vi "BLcompare.vi"(7 "Zref":dbl=500.0 min=0.0, 8 "Normalise?":bool=TRUE, 9 "aTarget":cluster{"Xvalues":dbl[], "Yvalues":dbl[]}={"Xvalues"=[0.75, 0.82, 0.85, 0.86, 0.9, 0.91, 0.94, 0.95, 0.96], "Yvalues"=[55.0, 75.0, 88.0, 122.0, 160.0, 220.0, 294.0, 385.0, 499.0]}, 10 "aSeries":cluster{"Xvalues":dbl[], "Yvalues":dbl[]}={"Xvalues"=[9.631456, 10.097028, 10.411531, 10.617216, 10.970124, 11.230059, 11.570385, 11.879879, 12.393209, 13.02907, 13.593284, 13.540779], "Yvalues"=[50.04624939, 67.04914093, 89.77313232, 120.27675629, 161.2066803, 216.03833008, 289.45019531, 387.77822876, 519.55065918, 696.23638916, 932.88671875, 1250.06018066]}) -> (0 "metric2value":dbl, 1 "metric2name":string, 2 "metric1value":dbl, 3 "metric1name":string)   [LabVIEW 2018]
uses:
  gnuplotScriptComponents/BLPlottersubVIs/Resampler.ctl
  <vilib>/Analysis/baseanly.llb/Mean (DBL).vi
  <vilib>/Analysis/5stat.llb/RMS (DBL).vi
  <vilib>/Analysis/NI_AALPro.lvlib
  <vilib>/Analysis/NI_AALBase.lvlib
panel:
  in  "BandHalfWidth(%)":dbl=0.05
  in  "Comparison":enum16{"PercentError", "PercentPointsInBand"}(ring)
  in  "milliseconds to wait":u32
  out "XY Graph":cluster{dbl[], dbl[]}[](graph)
  out "TargetResampled":cluster{"Xvalues":dbl[], "Yvalues":dbl[]}={"Xvalues"=[9.631456, 10.097028, 10.411531, 10.617216, 10.970124, 11.230059, 11.570385, 11.879879, 12.393209, 13.02907, 13.593284, 13.540779], "Yvalues"=[50.04624939, 67.04914093, 89.77313232, 120.27675629, 161.2066803, 216.03833008, 289.45019531, 387.77822876, 519.55065918, 696.23638916, 932.88671875, 1250.06018066]}
  out "aSeriesNormalised":cluster{"Xvalues":dbl[], "Yvalues":dbl[]}={"Xvalues"=[9.631456, 10.097028, 10.411531, 10.617216, 10.970124, 11.230059, 11.570385, 11.879879, 12.393209, 13.02907, 13.593284, 13.540779], "Yvalues"=[50.04624939, 67.04914093, 89.77313232, 120.27675629, 161.2066803, 216.03833008, 289.45019531, 387.77822876, 519.55065918, 696.23638916, 932.88671875, 1250.06018066]}
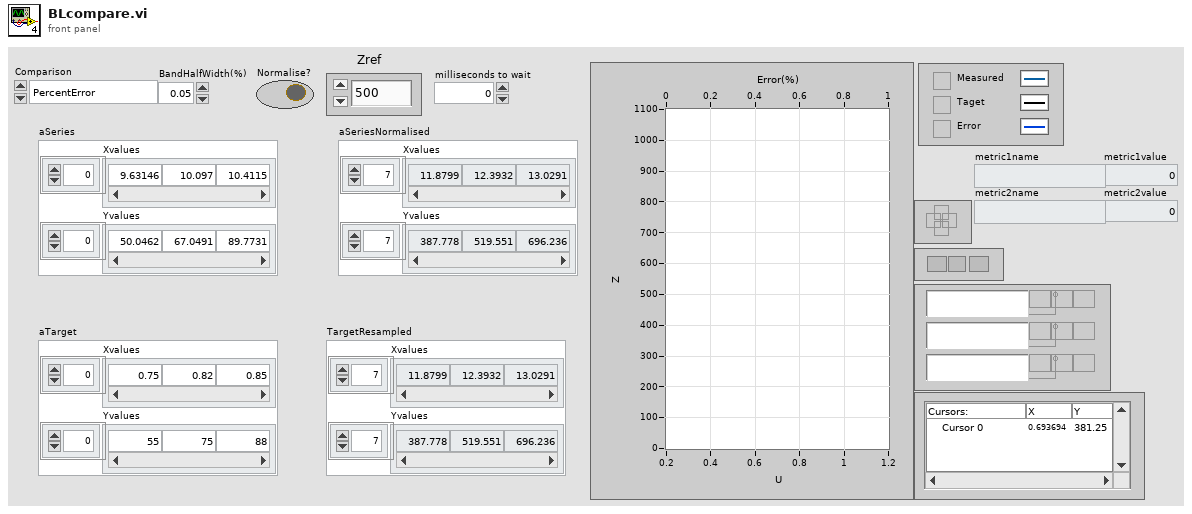
[diagram p1: front panel]
types:
  T1 = typedef "Resampler.ctl" = enum32{"AsTaken", "Regular", "Prescribed"}
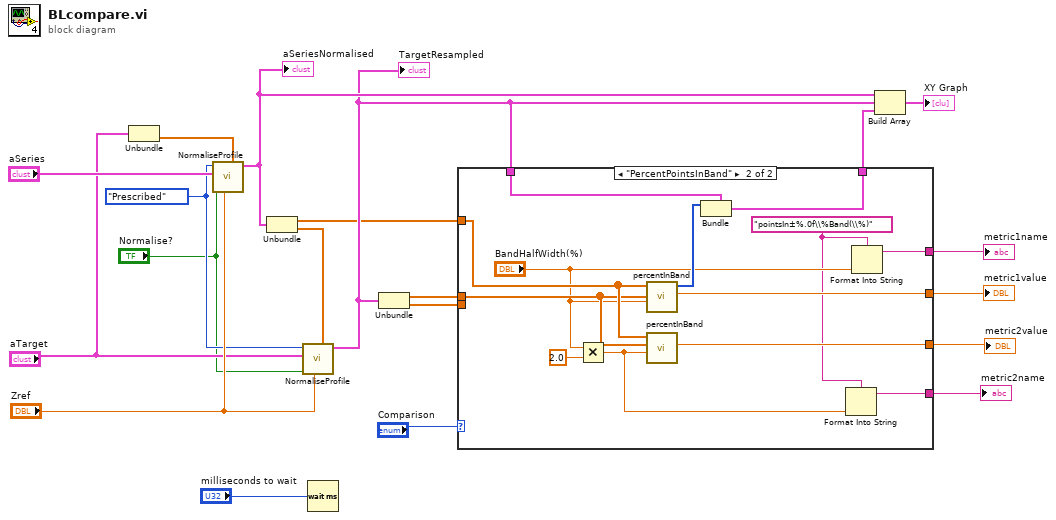
[diagram p0: block diagram]
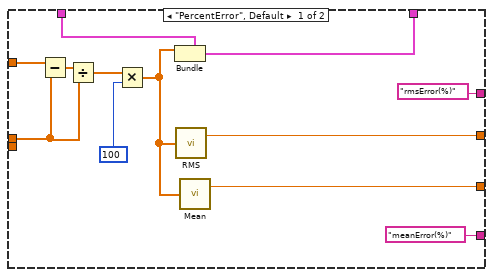
[diagram p2: hidden frame]
diagram:
  w15 = Resampler."Prescribed" ("Resampler")
  n1 = Unbundle("aTarget") -> ("Yvalues"=w16:dbl[])  [unwired: 1 out]
  n2 = call "NormaliseProfile.vi"("ResampleHeights"=w16, "Zref"="Zref", "Normalise?"="Normalise?", "UzClusterIn"="aSeries", "Resampler"=w15) -> ("UzClusterOutput"=w13:cluster{dbl[], dbl[]})  [unwired: 5 in, 1 out]
  "aSeriesNormalised" <- w13
  n3 = Unbundle(w13) -> (w9:dbl[], w19:dbl[])
  n4 = call "NormaliseProfile.vi"("ResampleHeights"=w19, "Zref"="Zref", "Normalise?"="Normalise?", "UzClusterIn"="aTarget", "Resampler"=w15) -> ("UzClusterOutput"=w12:cluster{dbl[], dbl[]})  [unwired: 5 in, 1 out]
  "TargetResampled" <- w12
  n5 = Wait (ms)(milliseconds to wait="milliseconds to wait") -> ()  [unwired: 1 out]
  n6 = Unbundle(w12) -> (w8:dbl[], w1:dbl[])
  n7 = case shown="\"PercentPointsInBand\"" "Comparison" {
    tunnel: w12 -> [w32 w45]
    tunnel: [w31 w44] -> w11
    tunnel: [w29 w43] -> w10
    tunnel: w9 -> [w26 w40]
    tunnel: w8 -> [w25 w39]
    tunnel: [w23 w36] -> w7
    tunnel: ["rmsError(%)" w41] -> w3
    tunnel: ["meanError(%)" w34] -> w4
    tunnel: w1 -> [_ _]
    frame "PercentError", Default {
      n8 = Subtract(x=w26, y=w25) -> (x-y=w30:dbl[])
      n9 = Divide(x=w30, y=w25) -> (x/y=w28:dbl[])
      n10 = Multiply(x=w28, y=100) -> (x*y=w24:dbl[])
      n11 = Bundle(cluster=w32, w24) -> (w31:cluster{dbl[], dbl[]})  [unwired: 1 in]
      n12 = call-poly <vilib>:"RMS.vi"("X"=w24) -> ("rms value"=w29:dbl)  [unwired: 1 out]
      n13 = call-poly <vilib>:"Mean.vi"("X"=w24) -> ("mean"=w23:dbl)  [unwired: 1 out]
    }
    frame "PercentPointsInBand" {
      w33 = "pointsIn±%.0f\\%Band(\\%)"
      n14 = Multiply(x="BandHalfWidth(%)", y=2.0) -> (x*y=w35:dbl)
      n15 = call "percentInBand.vi"("BandHalfWidth"="BandHalfWidth(%)", "targetPoints"=w39, "matchPoints"=w40) -> ("percentInBand"=w43:dbl, "inBand"=w42:i16[])  [unwired: 7 in]
      n16 = call "percentInBand.vi"("BandHalfWidth"=w35, "targetPoints"=w39, "matchPoints"=w40) -> ("percentInBand"=w36:dbl)  [unwired: 7 in, 1 out]
      n17 = Bundle(cluster=w45, w42) -> (w44:cluster{dbl[], dbl[]})  [unwired: 1 in]
      n18 = Format Into String(format string=w33, w35) -> (resulting string=w34:string)  [unwired: 2 in, 1 out]
      n19 = Format Into String(format string=w33, "BandHalfWidth(%)") -> (resulting string=w41:string)  [unwired: 2 in, 1 out]
    }
  }
  "metric1value" <- w10
  "metric2value" <- w7
  "metric2name" <- w4
  "metric1name" <- w3
  n20 = Build Array(w13, w12, w11) -> (→"XY Graph":cluster{dbl[], dbl[]}[])
